vi "Write Helper Loop.vi"(8 "error in (no error)":errorcluster, 10 "Helper Loop":refnum<class "Process.lvclass">, 11 "Helper Loop Test in":refnum<class "Helper Loop Test.lvclass">) -> (0 "error out":errorcluster, 3 "Helper Loop Test out":refnum<class "Helper Loop Test.lvclass">)   [LabVIEW 2020, in "Helper Loop Test.lvclass"]
uses:
  Helper Loop Test.lvclass
  Framework/Process/Process.lvclass
  Helper Loop Test.lvclass/Helper Loop Test.ctl
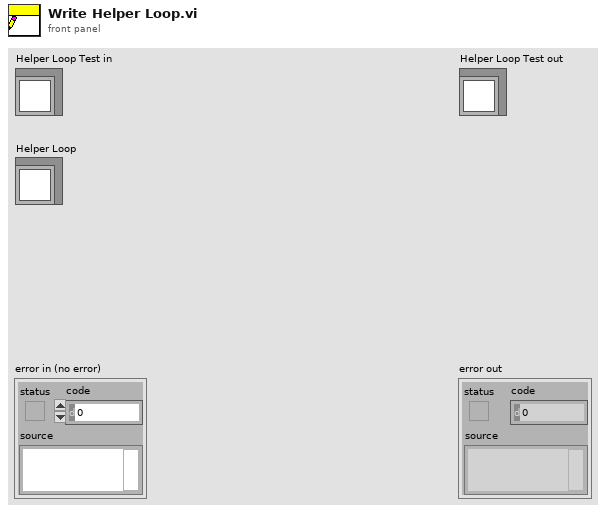
[diagram p1: front panel]
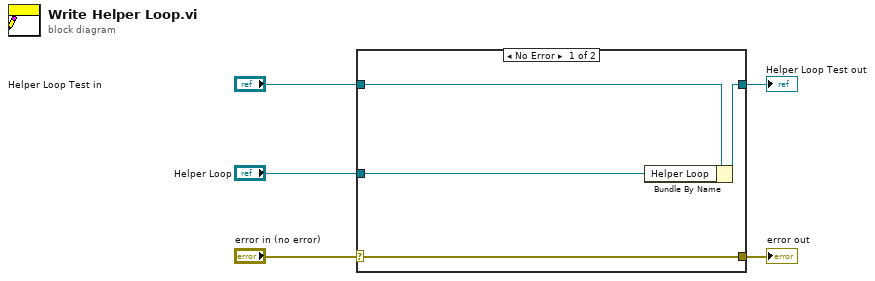
[diagram p0: block diagram]
diagram:
  n1 = case shown="No Error" "error in (no error)" {
    selector: "error in (no error)" -> [w9 w10]
    tunnel: [w9 w10] -> w4
    tunnel: [w7 w11] -> w2
    tunnel: "Helper Loop Test in" -> [w8 w11]
    tunnel: "Helper Loop" -> [w6 _]
    frame No Error {
      n2 = Bundle By Name(cluster=w8, "Helper Loop"=w6) -> (w7:refnum<class "Helper Loop Test.lvclass">)
    }
    frame Error {
    }
  }
  "error out" <- w4
  "Helper Loop Test out" <- w2
